vi "Get UTC from NTP_Flo_Test.vi"(8 "error in (no error)":errorcluster) -> (0 "error out":errorcluster, 3 "UTC Time":i64)   [LabVIEW 2014]
doc: "Gets the time using the NTP protocol and sets the RT clock to that time"
panel:
  out "Time Server\nUsed":string
  out "Time Server\nRequested":string
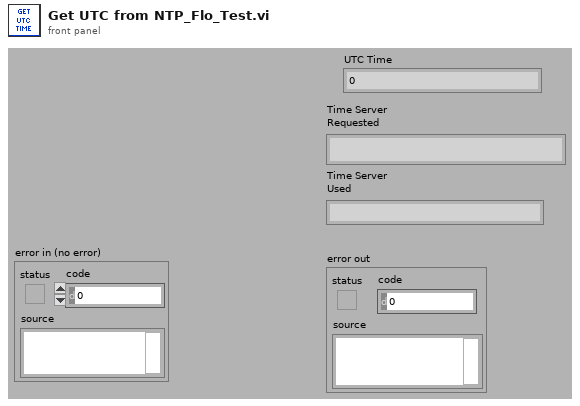
[diagram p1: front panel]
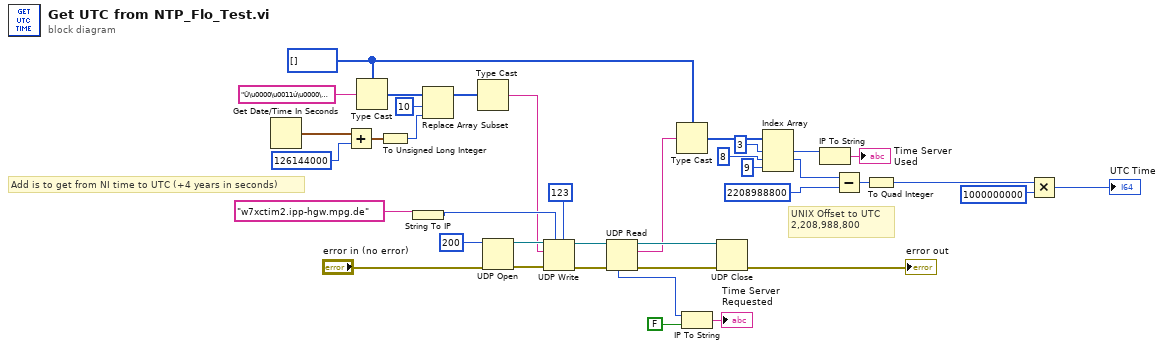
[diagram p0: block diagram]
diagram:
  w9 = i64[] []
  # "UNIX Offset to UTC\n2,208,988,800"
  # "Add is to get from NI time to UTC (+4 years in seconds)"
  n1 = Get Date/Time In Seconds() -> (seconds since 1Jan1904=w22:timestamp)
  n2 = Add(x=w22, y=u32 126144000) -> (x+y=w17:timestamp)
  n3 = Type Cast(type=w9, x="Û\u0000\u0011ú\u0000\u0000\u0000\u0000\u0000\u0001\u0003þ\u0000\u0000\u0000\u0000Ð!ú*\u0017KÆ§\u0000\u0000\u0000\u0000\u0000\u0000\u0000\u0000\u0000\u0000\u0000\u0000\u0000\u0000\u0000\u0000Ð'l\u001a‚MÒñ€:\u0000\u0000\u0000\u0000\u0000\u0000\u0000\u0000\u0000\u0000\u0000\u0000\u0000\u0000\u0000\u0000\u0000\u0000" ("String")) -> (*(type *) &x=w20:i64[])
  n4 = To Unsigned Long Integer(number=w17) -> (unsigned 32bit integer=w13:u32)
  n5 = String To IP(1:"w7xctim2.ipp-hgw.mpg.de" ("Time Server\nIP Address")) -> (0:w35:u32)
  n6 = Replace Array Subset(array=w20, new element=w13, index=10) -> (w19:i64[])
  n7 = Type Cast(x=w19) -> (*(type *) &x=w14:string)  [unwired: 1 in]
  n8 = UDP Open(8:"error in (no error)", 11:u16 200 ("port")) -> (port=w36:refnum<k16>, 0:w37:errorcluster)  [unwired: 3 in, 1 out]
  n9 = UDP Write(address=w35, port or service name=u16 123 ("port"), connection ID=w36, data in=w14, 8:w37) -> (error out=w34:errorcluster, 3:w33:refnum<k16>)  [unwired: 1 in]
  n10 = UDP Read(connection ID=w33, 8:w34) -> (data out=w25:string, error out=w31:errorcluster, 3:w32:refnum<k16>, 6:w28:u32)  [unwired: 2 in, 1 out]
  n11 = Type Cast(type=w9, x=w25) -> (*(type *) &x=w24:i64[])
  n12 = IP To String(1:FALSE ("dot notation? (F)"), 2:w28) -> (0:→"Time Server\nRequested":string)
  n13 = UDP Close(connection ID=w32, 8:w31) -> (error out=→"error out":errorcluster)  [unwired: 1 out]
  n14 = Index Array(array=w24, index #1=3 ("index"), index #2=8 ("index"), index #3=9 ("index")) -> (element #1=w12:i64, element #2=w6:i64)  [unwired: 1 out]
  n15 = IP To String(2:w12) -> (0:→"Time Server\nUsed":string)  [unwired: 1 in]
  n16 = Subtract(x=w6, y=i64 2208988800) -> (x-y=w4:i64)
  n17 = To Quad Integer(1:w4) -> (0:w1:i64)
  n18 = Multiply(x=w1, y=i64 1000000000 ("lo")) -> (x*y=→"UTC Time":i64)
